vi "Wait For CMD Ack.vi"(5 "Timeout":u16, 6 "Mdrive Mode":T1=enum."Party Mode", 7 "Device Name":string, 8 "error in (no error)":errorcluster, 9 "Get Parameter":T2, 10 "ExpectedValue":i32, 11 "VISA Refnum in":refnum<visa-resource-name>) -> (0 "error out":errorcluster, 3 "VISA Refnum out":refnum<visa-resource-name>)   [LabVIEW 2015]
uses:
  MCode_LV_86/Get Parameter.ctl
  MCode_LV_86/MDrive Mode.ctl
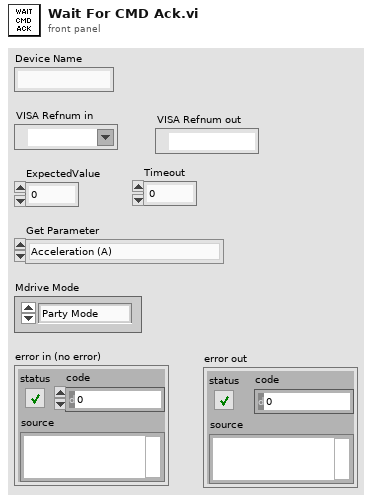
[diagram p1: front panel]
types:
  T1 = typedef "MDrive Mode.ctl" = enum16{"Normal Mode", "Party Mode"}
  T2 = typedef "Get Parameter.ctl" = enum16{"Acceleration (A)", "Baud Rate (BD)", "Busy Flag (BY)", "Counter 1 (C1)", "Counter 2 (C2)", "Check Sum Enable (CK)", "Clock Mode (CM)", "Clock Mode Ratio (CR)", "Clock Mode Out Step Width (CW)", "Deceleration (D)", "Digital Filtering, Input 1 (D1)", "Digital Filtering, Input 2 (D2)", "Digital Filtering, Input 3 (D3)", "Digital Filtering, Input 4 (D4)", "Digital Filtering, Input 5 (D5)", "Digital Filtering, Input 9 (D9)", "Digital Filtering, Input 10 (D10)", "Digital Filtering, Input 11 (D11)", "Digital Filtering, Input 12 (D12)", "Deadband (DB)", "Enable/Disable Drive (DE)", "Device Name (DN)", "End Program Execution (E)", "Encoder Function Enable (EE)", "Encoder Lines (EL)", "Error Flag (EF)", "Error Variable (ER)", "Echo Mode (EM)", "Escape (ES)", "Execute Program at Address (EX)", "Hold Current (HC)", "Hold Current Delay Time (HI)", "Input 1 (I1)", "Input 2 (I2)", "Input 3 (I3)", "Input 4 (I4)", "Input 5 Analog (I5)", "Input 6 Encoder Index (I6)", "Input 9 (I9)", "Input 10 (I10)", "Input 11 (I11)", "Input 12 (I12)", "Input Low Byte (1-4) (IL)", "Input High Byte (9-12) (IH)", "Inputs Total (1-4,9-12) (IN)", "Internal Temperature (IT)", "Jog Enable (JE)", "Limit Stop Mode (LM)", "MicroStepping Select (MS)", "Motor Settling Delay Time (MT)", "Moving Flag (MV)", "Output 1 (O1)", "Output 2 (O2)", "Output 3 (O3)", "Output 4 (O4)", "Output 9 (O9)", "Output 10 (O10)", "Output 11 (O11)", "Output 12 (O12)", "Output High Byte (9-12) (OH)", "Output Low Byte (1-4) (OL)", "Output Total (1-4 and 9-12) (OT)", "Position (P)", "Position Captured at Trip (PC)", "Position Maintenance (PM)", "Part Number (PN)", "Party Mode (PY)", "Register 1 (R1)", "Register 2 (R2)", "Register 3 (R3)", "Register 4 (R4)", "Run Current (RC)", "Serial Number (SN)", "Stall Flag (ST)", "Stall Factor (SF)", "Stall Mode Set (SM)", "User Variables (UV)", "Velocity (V)", "Velocity Changing Flag (VC)", "Velocity Initial (VI)", "Version, Firmware (VR)", "Velocity Maximum (VM)", "Read Input1", "Read Input2"}
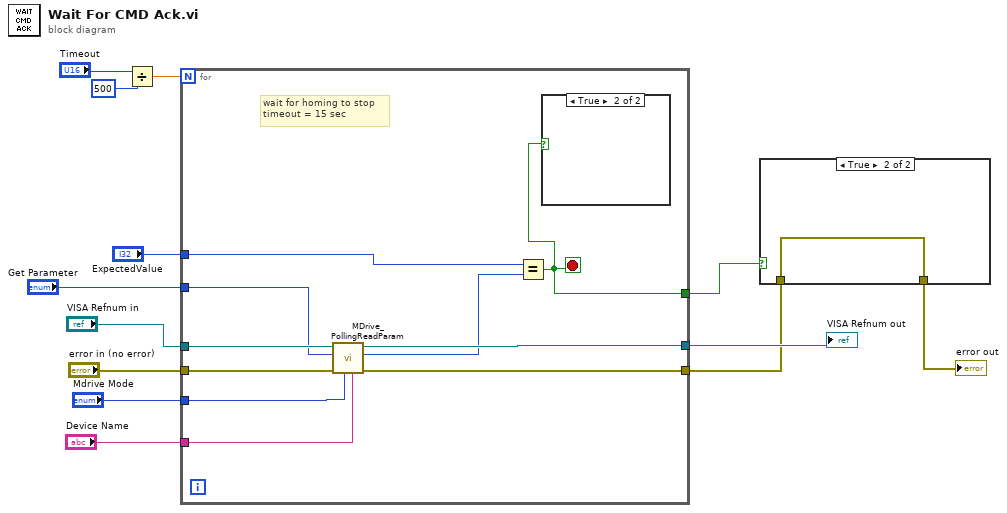
[diagram p0: block diagram]
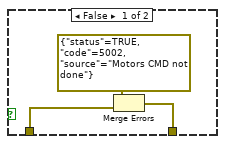
[diagram p2: hidden frame]
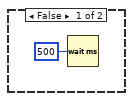
[diagram p3: hidden frame]
diagram:
  n1 = Divide(x="Timeout", y=u16 500) -> (x/y=w5:dbl)
  n2 = for {
    N: w5 -> [_]
    tunnel: [w23] -> w2
    tunnel: [w22] -> w4
    tunnel: [w21] -> w3
    tunnel: "VISA Refnum in" -> [w20]
    tunnel: "error in (no error)" -> [w19]
    tunnel: "Mdrive Mode" -> [w18]
    tunnel: "Device Name" -> [w17]
    tunnel: "ExpectedValue" -> [w15]
    tunnel: "Get Parameter" -> [w14]
    stop <- w21 stop-if-true
    # "wait for homing to stop\ntimeout = 15 sec"
    n3 = call "MDrive_PollingReadParam.vi"("Device Name"=w17, "Mdrive Mode"=w18, "error in (no error)"=w19, "Get Parameter"=w14, "VISA Refnum in"=w20) -> ("error out"=w23:errorcluster, "Value"=w16:i32, "VISA Refnum out"=w22:refnum<visa-resource-name>)  [unwired: 3 in, 1 out]
    n4 = Equal?(x=w15, y=w16) -> (x = y?=w21:bool)
    n5 = case shown="True" w21 {
      frame False {
        n6 = Wait (ms)(milliseconds to wait=u32 500) -> ()  [unwired: 1 out]
      }
      frame True {
      }
    }
  }
  "VISA Refnum out" <- w4
  n7 = case shown="True" w3 {
    tunnel: w2 -> [w27 w28]
    tunnel: [w26 w28] -> w1
    frame False {
      n8 = Merge Errors(errorcluster {"status"=TRUE, "code"=5002, "source"="Motors CMD not done"} ("error in"), w27) -> (w26:errorcluster)
    }
    frame True {
    }
  }
  "error out" <- w1
